vi "Scanning Motion One Direction for Y Multiple Readings per Point With Phase Info.vi"() -> ()   [LabVIEW 2021]
uses:
  <vilib>/Utility/file.llb/Write Delimited Spreadsheet (DBL).vi
  MID-main/Marlin Instrument Driver/Marlin Instrument Driver.lvlib
  <instrlib>/Siglent SDS 1000 2000 Series/Siglent SDS 1000 2000 Series.lvlib
panel:
  in  "Samples per pt":dbl=5.0
  in  "VISA resource name o-scope":refnum<visa-resource-name>="USB0::0xF4ED::0xEE3A::SDS1EDED5R2476::INSTR"
  in  "Measurement (0: Vpp)":u16(ring) items=["Vpp", "Vmax", "Vmin", "Vamp", "Vtop", "Vbase", "Vavg", "Mean", "Vrms", "Crms", "FOV", "FPRE", "ROV", "RPRE", "Period", "Freq", "+Wid", "-Wid", "Rise Time", "Fall Time", "Bwid", "+Duty", "-Duty"]
  in  "Source (1: Channel 1)":u16(ring)=1 items=["Channel 1"=1, "Channel 2"=2, "Channel 3"=3, "Channel 4"=4]
  in  "file path (dialog if empty)":path=path "C:/Users/scoughen/Documents/Printer Controll/Coughenour Programs/Scan Data/LiLens500kHzHighResPhaseScanOrthogonal5SampleAvg0SecDelay3mmOffsetFromTransducerNewAmp9.6Vpp.csv"
  in  "T":dbl
  in  "y Flag":string="Negative"
  in  "x Flag":string="Negative"
  in  "linearF":dbl=1000.0
  in  "E":dbl
  in  "rapidF":dbl=3000.0
  in  "zRes":dbl=0.5
  in  "yRes":dbl=0.5
  in  "xRes":dbl=1.0
  in  "zSize":dbl=80.0
  in  "ySize":dbl=50.0
  in  "xSize":dbl=5.0
  in  "zInit":dbl=149.0
  in  "yInit":dbl=188.0
  in  "xInit":dbl=87.0
  out "error out":errorcluster
  in  "error in (no error)":errorcluster
  in  "VISA resource name":refnum<visa-resource-name>="COM5"
  # "All Units in mm"
  # "Initial Position"
  # "Scan Size"
  # "Scan Resolution"
  # "Extrusion"
  # "Feed Rate"
  # "Read Delay (s)"
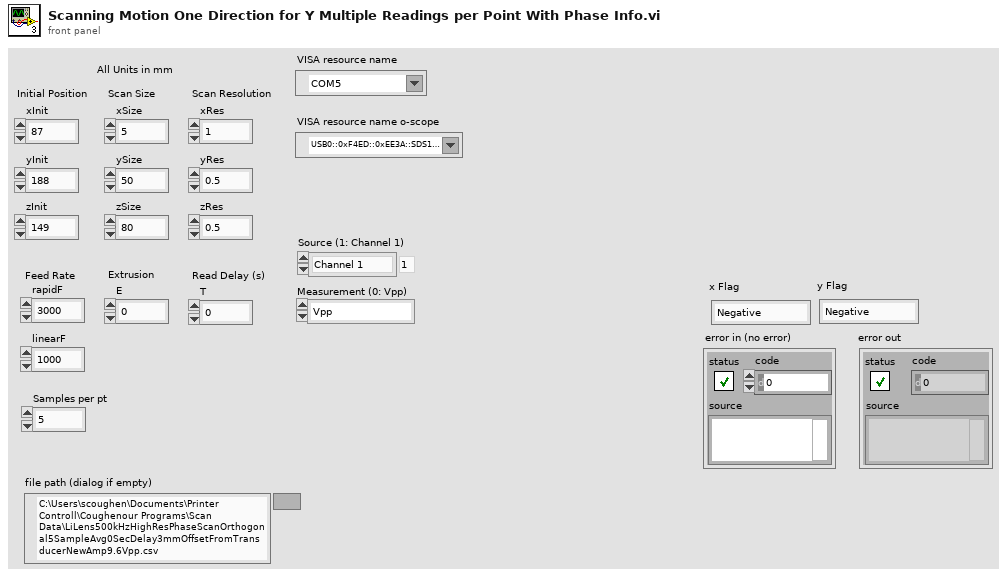
[diagram p1: front panel]
types:
  T1 = cluster{"E":dbl, "rapidF":dbl, "xInit":dbl, "yInit":dbl, "zInit":dbl}
  T2 = cluster{"E":dbl, "linearF":dbl, dbl, "yInit":dbl, "zInit":dbl}
  T3 = cluster{"E":dbl, "linearF":dbl, "xInit":dbl, dbl, "zInit":dbl}
  T4 = cluster{"E":dbl, "linearF":dbl, dbl, "zInit":dbl, "yInit":dbl}
  T5 = cluster{"E":dbl, "linearF":dbl, "xInit":dbl, "yInit":dbl, dbl}
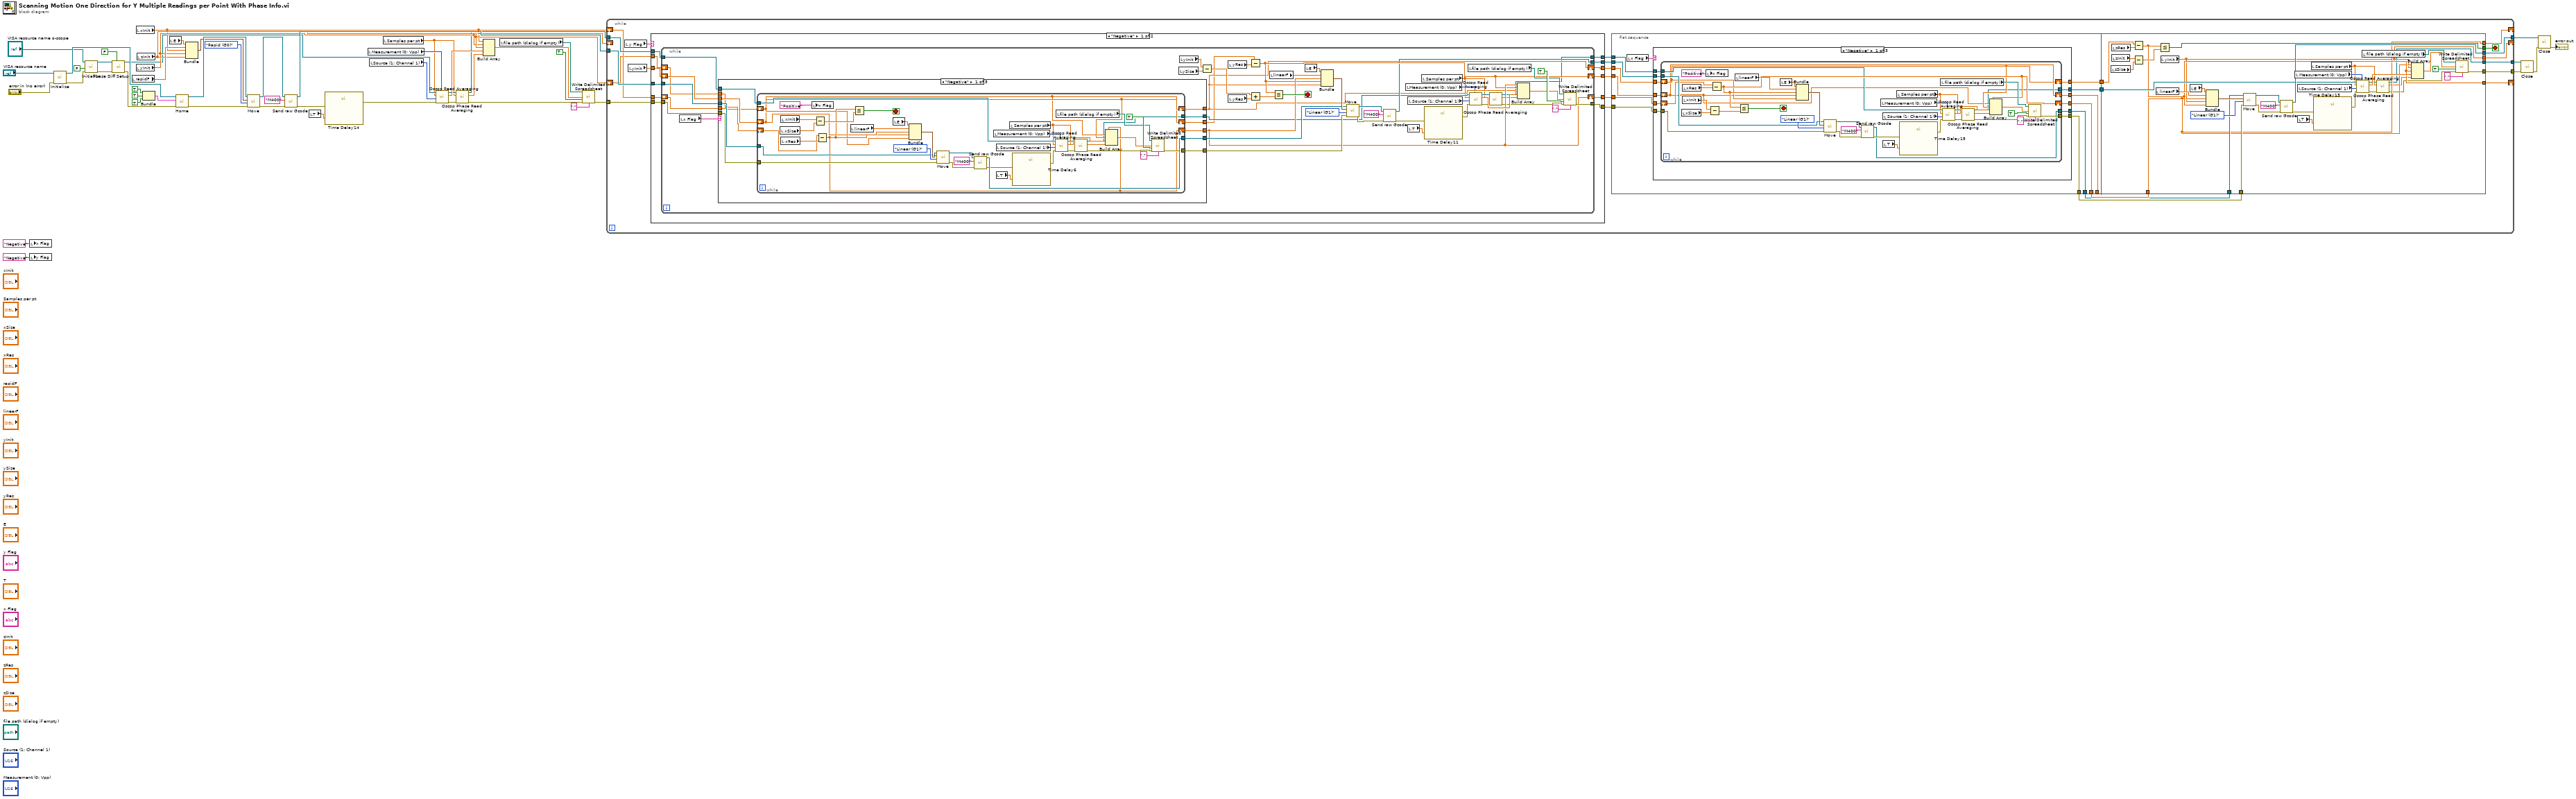
[diagram p0: block diagram]
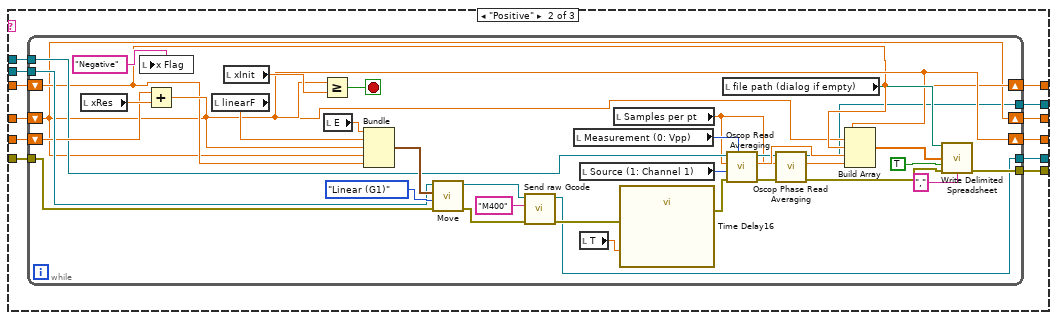
[diagram p2: hidden frame]
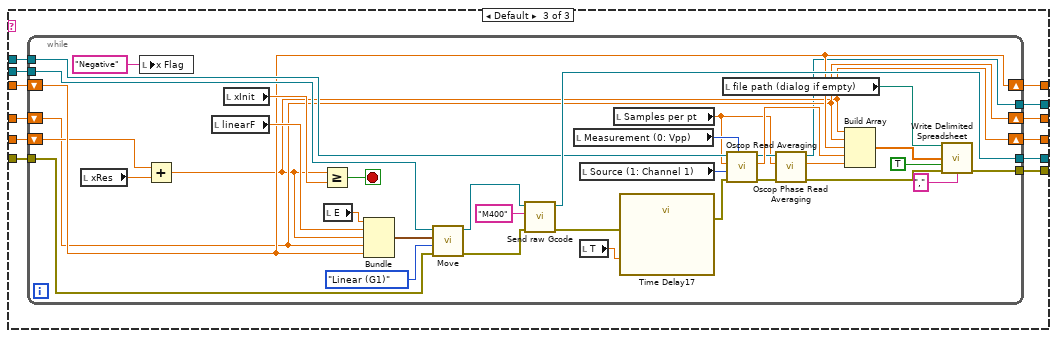
[diagram p3: hidden frame]
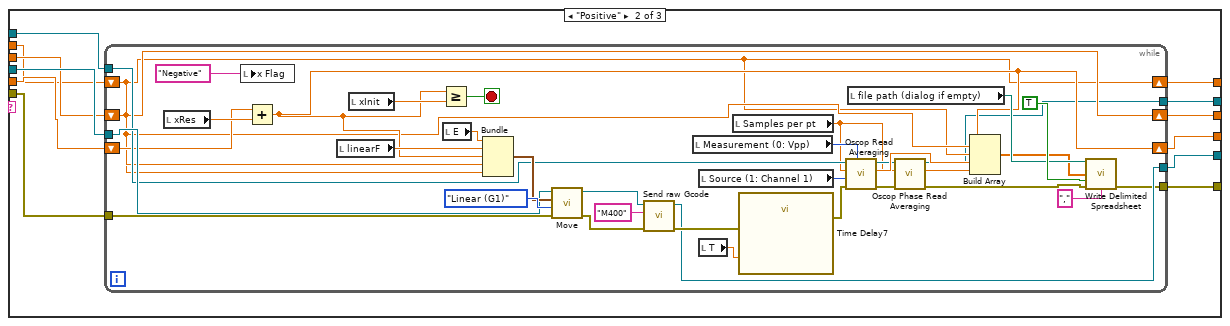
[diagram p4: hidden frame]
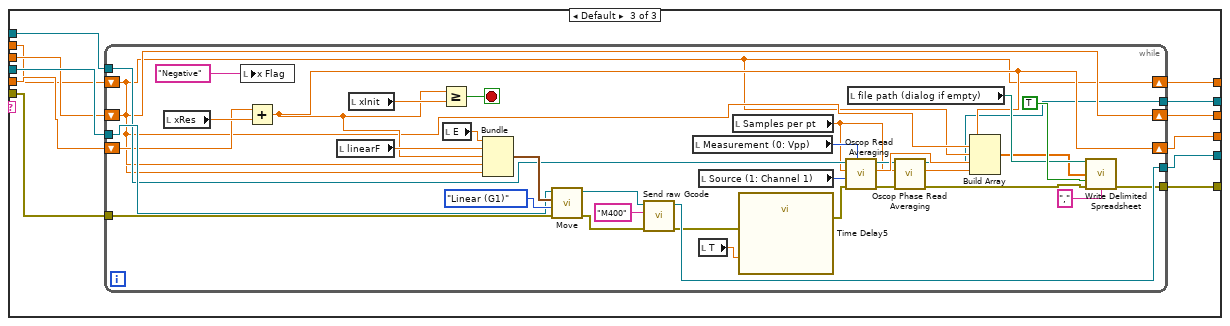
[diagram p5: hidden frame]
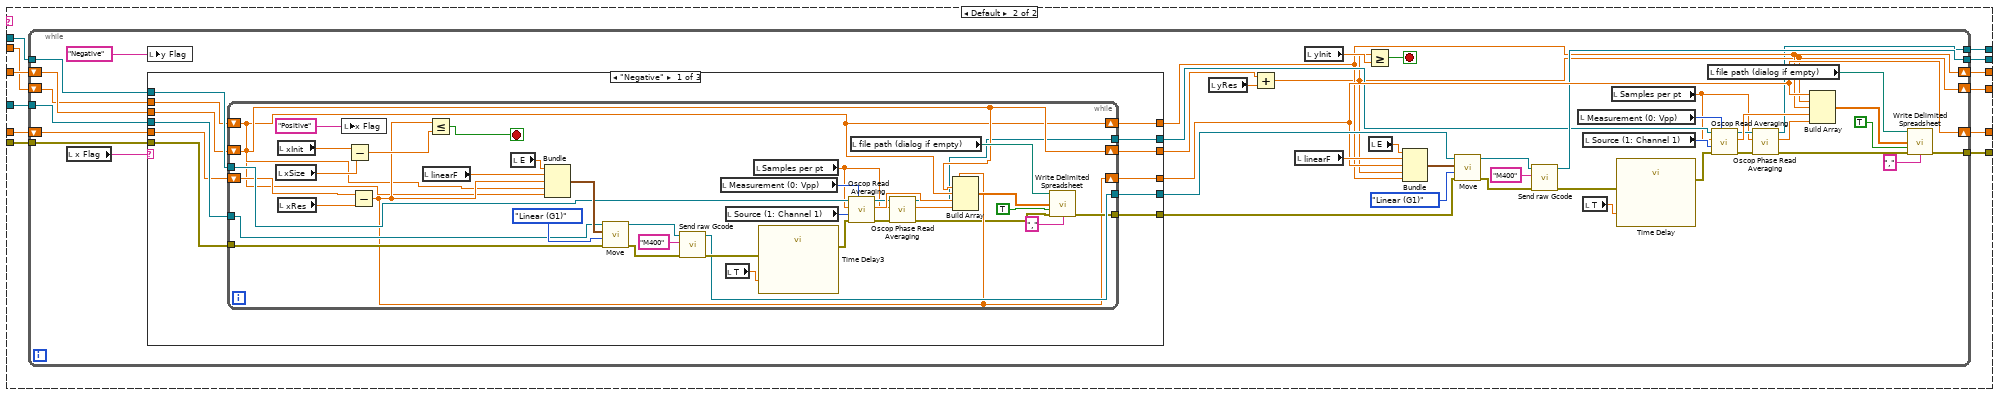
[diagram p6: hidden frame]
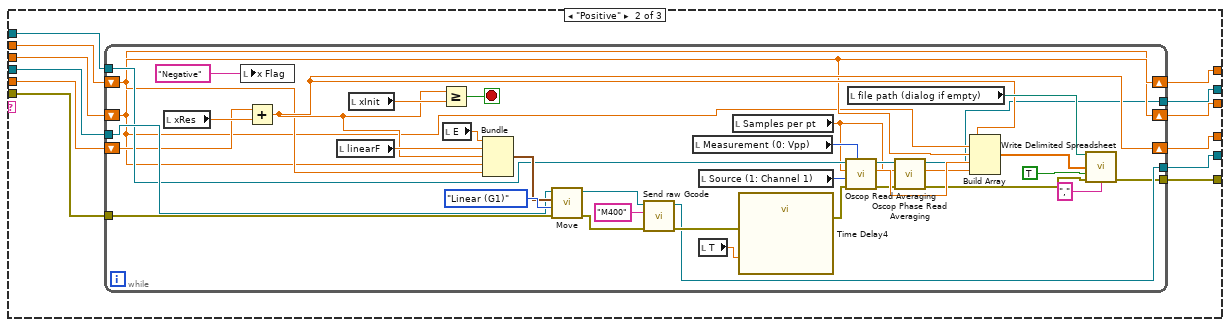
[diagram p7: hidden frame]
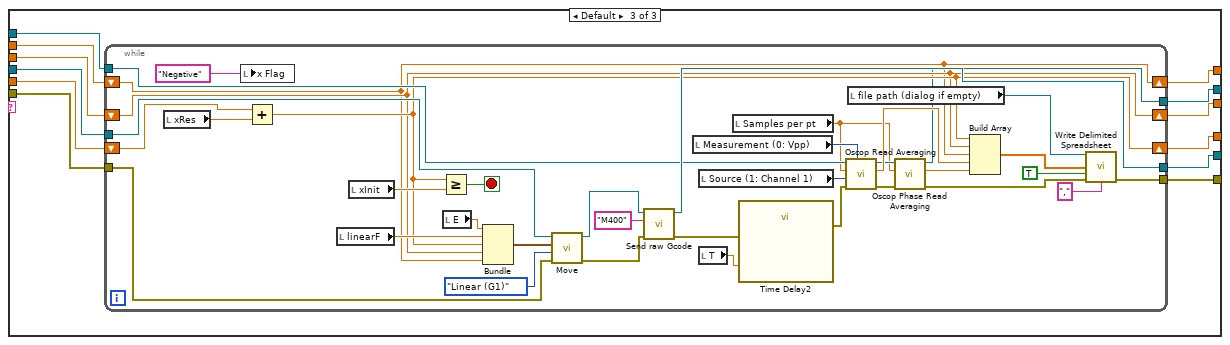
[diagram p8: hidden frame]
diagram:
  n1 = local write "x Flag"("Negative" ("x Flag")) -> ()
  n2 = local write "y Flag"("Negative" ("y Flag")) -> ()
  n3 = call <instrlib>:"Initialize.vi"("error in (no error)"="error in (no error)", "VISA resource name"="VISA resource name") -> ("error out"=w29:errorcluster, "VISA resource name out"=w49:refnum<visa-resource-name>)  [unwired: 8 in]
  n4 = call <instrlib>:"Initialize.vi"("error in (no error)"=w29, "Reset (True)"=FALSE, "VISA resource name"="VISA resource name o-scope") -> ("error out"=w6:errorcluster, "VISA resource name out"=w4:refnum<visa-resource-name>)  [unwired: 7 in]
  n5 = call "Phase Diff Setup.vi"("Perform Auto Setup"=FALSE, "error in (no error)"=w6, "VISA resource name"=w4) -> ("error out"=w5:errorcluster, "VISA resource name out"=w3:refnum<visa-resource-name>)  [unwired: 7 in]
  n6 = local read "rapidF"() -> (w39:dbl)
  n7 = local read "xInit"() -> (w16:dbl)
  n8 = local read "yInit"() -> (w17:dbl)
  n9 = local read "zInit"() -> (w18:dbl)
  n10 = Bundle(TRUE, TRUE, TRUE) -> (w45:cluster{bool, bool, bool})  [unwired: 1 in]
  n11 = local read "E"() -> (w38:dbl)
  n12 = call "Home.vi"("error in (no error)"=w5, "Axes"=w45, "VISA resource name"=w49) -> ("error out"=w44:errorcluster, "VISA resource name out"=w43:refnum<visa-resource-name>)  [unwired: 7 in]
  n13 = Bundle("E"=w38, "rapidF"=w39, "xInit"=w16, "yInit"=w17, "zInit"=w18) -> (w41:T1)  [unwired: 1 in]
  n14 = call "Move.vi"("error in (no error)"=w44, "type"=enum16{"Rapid (G0)", "Linear (G1)"}."Rapid (G0)" ("type 2"), "Distances"=w41, "VISA resource name"=w43) -> ("error out"=w33:errorcluster, "VISA resource name out"=w34:refnum<visa-resource-name>)  [unwired: 6 in]
  n15 = call "Send raw Gcode.vi"("error in (no error)"=w33, "Gcode"="M400", "VISA resource name"=w34) -> ("error out"=w31:errorcluster, "VISA resource name out"=w32:refnum<visa-resource-name>)  [unwired: 5 in, 2 out]
  n16 = local read "T"() -> (w35:dbl)
  n17 = call "Time Delay14"("error in (no error)"=w31, "Delay Time (s)"=w35) -> ("error out"=w21:errorcluster)  [unwired: 9 in]
  n18 = local read "Measurement (0: Vpp)"() -> (w12:u16)
  n19 = local read "Source (1: Channel 1)"() -> (w19:u16)
  n20 = local read "Samples per pt"() -> (w1:dbl)
  n21 = call "Oscop Read Averaging.vi"("Measurement (0: Vpp)"=w12, "error in (no error)"=w21, "Source (1: Channel 1)"=w19, "Numeric in"=w1, "VISA Refnum in"=w3) -> ("error out"=w9:errorcluster, "Numeric out"=w13:dbl, "VISA Refnum out"=w8:refnum<visa-resource-name>)  [unwired: 4 in]
  n22 = call "Oscop Phase Read Averaging.vi"("error in (no error)"=w9, "Numeric in"=w1, "VISA Refnum in"=w8) -> ("error out"=w10:errorcluster, "Numeric out"=w7:dbl, "VISA Refnum out"=w11:refnum<visa-resource-name>)  [unwired: 6 in]
  n23 = Build Array(w16, w17, w18, w13, w7) -> (w22:dbl[])
  n24 = local read "file path (dialog if empty)"() -> (w15:path)
  n25 = call-poly <vilib>:"Write Delimited Spreadsheet.vi"("file path (dialog if empty)"=w15, "1D data"=w22, "append to file? (new file:F)"=TRUE, "error in (no error)"=w10, "delimiter (\\t)"="," ("delimiter (\\t)")) -> ("error out"=w20:errorcluster)  [unwired: 9 in, 1 out]
  n26 = while {
    tunnel: w32 -> [w77]
    tunnel: w20 -> [w76]
    tunnel: [w67] -> w40
    tunnel: [w66] -> w27
    tunnel: [w64] -> w25
    tunnel: w11 -> [w61]
    shift-right: [w56] -> _
    shift-left: w18 -> [w59]
    shift-right: [w55] -> _
    shift-left: w17 -> [_]
    shift-right: [w54] -> _
    shift-left: w16 -> [w60]
    stop <- w65 stop-if-true
    n27 = local read "y Flag"() -> (w75:string)
    n28 = local read "yInit"() -> (w53:dbl)
    n29 = case shown="\"Negative\"" w75 {
      tunnel: w77 -> [w285 w489]
      tunnel: [w282 w488] -> w74
      tunnel: w76 -> [w284 w487]
      tunnel: [w283 w486] -> w73
      tunnel: [w281 w485] -> w71
      tunnel: [w280 w484] -> w72
      tunnel: [w279 w483] -> w58
      tunnel: [w278 w482] -> w62
      tunnel: w61 -> [w277 w481]
      tunnel: w60 -> [w275 w478]
      tunnel: w53 -> [w276 w480]
      tunnel: w59 -> [w274 w479]
      frame "Negative" {
        n30 = while {
          tunnel: w285 -> [w329]
          tunnel: [w300] -> w282
          tunnel: w284 -> [w327]
          tunnel: [w303] -> w283
          tunnel: [w290] -> w278
          tunnel: w277 -> [w298]
          shift-right: [w301] -> w280
          shift-left: w276 -> [w295]
          shift-right: [w302] -> w281
          shift-left: w275 -> [w294]
          shift-right: [w297] -> w279
          shift-left: w274 -> [w293]
          stop <- w325 stop-if-true
          n31 = local read "x Flag"() -> (w324:string)
          n32 = case shown="\"Negative\"" w324 {
            tunnel: w329 -> [w343 w393 w441]
            tunnel: [w340 w392 w440] -> w328
            tunnel: w327 -> [w342 w391 w439]
            tunnel: [w341 w390 w437] -> w326
            tunnel: [w339 w389 w438] -> w302
            tunnel: [w338 w388 w436] -> w296
            tunnel: [w336 w387 w434] -> w299
            tunnel: w298 -> [w337 w386 w435]
            tunnel: w294 -> [w335 w385 w433]
            tunnel: w295 -> [w334 w384 w432]
            tunnel: w293 -> [w332 w383 w431]
            tunnel: [w333 w382 w430] -> w297
            frame "Negative" {
              n33 = while {
                tunnel: w343 -> [w379]
                tunnel: [w366] -> w340
                tunnel: w342 -> [w378]
                tunnel: [w357] -> w341
                tunnel: w337 -> [w356]
                tunnel: [w348] -> w336
                shift-right: [w354] -> w339
                shift-left: w335 -> [w355]
                shift-right: [w352] -> w338
                shift-left: w334 -> [w352]
                shift-right: [w353] -> w333
                shift-left: w332 -> [w353]
                stop <- w377 stop-if-true
                n34 = local read "xSize"() -> (w371:dbl)
                n35 = local read "xInit"() -> (w372:dbl)
                n36 = local read "xRes"() -> (w374:dbl)
                n37 = local write "x Flag"("Positive" ("x Flag")) -> ()
                n38 = Subtract(x=w372, y=w371) -> (x-y=w370:dbl)
                n39 = Subtract(x=w355, y=w374) -> (x-y=w354:dbl)
                n40 = local read "linearF"() -> (w375:dbl)
                n41 = Less Or Equal?(x=w354, y=w370) -> (x <= y?=w377:bool)
                n42 = local read "E"() -> (w376:dbl)
                n43 = Bundle("E"=w376, "linearF"=w375, w354, "yInit"=w352, "zInit"=w353) -> (w380:T2)  [unwired: 1 in]
                n44 = call "Move.vi"("error in (no error)"=w378, "type"=enum16{"Rapid (G0)", "Linear (G1)"}."Linear (G1)" ("type 2"), "Distances"=w380, "VISA resource name"=w379) -> ("error out"=w365:errorcluster, "VISA resource name out"=w367:refnum<visa-resource-name>)  [unwired: 6 in]
                n45 = call "Send raw Gcode.vi"("error in (no error)"=w365, "Gcode"="M400", "VISA resource name"=w367) -> ("error out"=w364:errorcluster, "VISA resource name out"=w366:refnum<visa-resource-name>)  [unwired: 5 in, 2 out]
                n46 = local read "Measurement (0: Vpp)"() -> (w350:u16)
                n47 = local read "Source (1: Channel 1)"() -> (w351:u16)
                n48 = local read "T"() -> (w369:dbl)
                n49 = local read "Samples per pt"() -> (w344:dbl)
                n50 = call "Time Delay6"("error in (no error)"=w364, "Delay Time (s)"=w369) -> ("error out"=w358:errorcluster)  [unwired: 9 in]
                n51 = call "Oscop Read Averaging.vi"("Measurement (0: Vpp)"=w350, "error in (no error)"=w358, "Source (1: Channel 1)"=w351, "Numeric in"=w344, "VISA Refnum in"=w356) -> ("error out"=w345:errorcluster, "Numeric out"=w359:dbl, "VISA Refnum out"=w346:refnum<visa-resource-name>)  [unwired: 4 in]
                n52 = local read "file path (dialog if empty)"() -> (w361:path)
                n53 = call "Oscop Phase Read Averaging.vi"("error in (no error)"=w345, "Numeric in"=w344, "VISA Refnum in"=w346) -> ("error out"=w349:errorcluster, "Numeric out"=w347:dbl, "VISA Refnum out"=w348:refnum<visa-resource-name>)  [unwired: 6 in]
                n54 = Build Array(w354, w352, w353, w359, w347) -> (w360:dbl[])
                n55 = call-poly <vilib>:"Write Delimited Spreadsheet.vi"("file path (dialog if empty)"=w361, "1D data"=w360, "append to file? (new file:F)"=TRUE, "error in (no error)"=w349, "delimiter (\\t)"="," ("delimiter (\\t)")) -> ("error out"=w357:errorcluster)  [unwired: 9 in, 1 out]
              }
            }
            frame "Positive" {
              n56 = while {
                tunnel: w393 -> [w427]
                tunnel: [w414] -> w392
                tunnel: w391 -> [w426]
                tunnel: [w407] -> w390
                tunnel: [w398] -> w387
                tunnel: w386 -> [w405]
                shift-right: [w406] -> w389
                shift-left: w385 -> [w404]
                shift-right: [w403] -> w388
                shift-left: w384 -> [w403]
                shift-right: [w402] -> w382
                shift-left: w383 -> [w402]
                stop <- w425 stop-if-true
                n57 = local read "xRes"() -> (w423:dbl)
                n58 = local write "x Flag"("Negative" ("x Flag")) -> ()
                n59 = Add(x=w404, y=w423) -> (x+y=w406:dbl)
                n60 = local read "linearF"() -> (w422:dbl)
                n61 = local read "xInit"() -> (w424:dbl)
                n62 = Greater Or Equal?(x=w406, y=w424) -> (x >= y?=w425:bool)
                n63 = local read "E"() -> (w421:dbl)
                n64 = Bundle("E"=w421, "linearF"=w422, w406, "yInit"=w403, "zInit"=w402) -> (w428:T2)  [unwired: 1 in]
                n65 = call "Move.vi"("error in (no error)"=w426, "type"=enum16{"Rapid (G0)", "Linear (G1)"}."Linear (G1)" ("type 2"), "Distances"=w428, "VISA resource name"=w427) -> ("error out"=w417:errorcluster, "VISA resource name out"=w415:refnum<visa-resource-name>)  [unwired: 6 in]
                n66 = call "Send raw Gcode.vi"("error in (no error)"=w417, "Gcode"="M400", "VISA resource name"=w415) -> ("error out"=w416:errorcluster, "VISA resource name out"=w414:refnum<visa-resource-name>)  [unwired: 5 in, 2 out]
                n67 = local read "Measurement (0: Vpp)"() -> (w400:u16)
                n68 = local read "Source (1: Channel 1)"() -> (w401:u16)
                n69 = local read "T"() -> (w419:dbl)
                n70 = local read "Samples per pt"() -> (w394:dbl)
                n71 = call "Time Delay7"("error in (no error)"=w416, "Delay Time (s)"=w419) -> ("error out"=w408:errorcluster)  [unwired: 9 in]
                n72 = call "Oscop Read Averaging.vi"("Measurement (0: Vpp)"=w400, "error in (no error)"=w408, "Source (1: Channel 1)"=w401, "Numeric in"=w394, "VISA Refnum in"=w405) -> ("error out"=w396:errorcluster, "Numeric out"=w409:dbl, "VISA Refnum out"=w397:refnum<visa-resource-name>)  [unwired: 4 in]
                n73 = local read "file path (dialog if empty)"() -> (w411:path)
                n74 = call "Oscop Phase Read Averaging.vi"("error in (no error)"=w396, "Numeric in"=w394, "VISA Refnum in"=w397) -> ("error out"=w399:errorcluster, "Numeric out"=w395:dbl, "VISA Refnum out"=w398:refnum<visa-resource-name>)  [unwired: 6 in]
                n75 = Build Array(w406, w403, w402, w409, w395) -> (w410:dbl[])
                n76 = call-poly <vilib>:"Write Delimited Spreadsheet.vi"("file path (dialog if empty)"=w411, "1D data"=w410, "append to file? (new file:F)"=TRUE, "error in (no error)"=w399, "delimiter (\\t)"="," ("delimiter (\\t)")) -> ("error out"=w407:errorcluster)  [unwired: 9 in, 1 out]
              }
            }
            frame Default {
              n77 = while {
                tunnel: w441 -> [w475]
                tunnel: [w464] -> w440
                tunnel: w439 -> [w474]
                tunnel: [w455] -> w437
                tunnel: w435 -> [w454]
                tunnel: [w446] -> w434
                shift-right: [w453] -> w438
                shift-left: w433 -> [w452]
                shift-right: [w451] -> w436
                shift-left: w432 -> [w451]
                shift-right: [w450] -> w430
                shift-left: w431 -> [w450]
                stop <- w473 stop-if-true
                n78 = local read "xRes"() -> (w471:dbl)
                n79 = local write "x Flag"("Negative" ("x Flag")) -> ()
                n80 = Add(x=w452, y=w471) -> (x+y=w453:dbl)
                n81 = local read "linearF"() -> (w470:dbl)
                n82 = local read "xInit"() -> (w472:dbl)
                n83 = Greater Or Equal?(x=w453, y=w472) -> (x >= y?=w473:bool)
                n84 = local read "E"() -> (w469:dbl)
                n85 = Bundle("E"=w469, "linearF"=w470, w453, "yInit"=w451, "zInit"=w450) -> (w476:T2)  [unwired: 1 in]
                n86 = call "Move.vi"("error in (no error)"=w474, "type"=enum16{"Rapid (G0)", "Linear (G1)"}."Linear (G1)" ("type 2"), "Distances"=w476, "VISA resource name"=w475) -> ("error out"=w463:errorcluster, "VISA resource name out"=w465:refnum<visa-resource-name>)  [unwired: 6 in]
                n87 = call "Send raw Gcode.vi"("error in (no error)"=w463, "Gcode"="M400", "VISA resource name"=w465) -> ("error out"=w462:errorcluster, "VISA resource name out"=w464:refnum<visa-resource-name>)  [unwired: 5 in, 2 out]
                n88 = local read "Measurement (0: Vpp)"() -> (w448:u16)
                n89 = local read "Source (1: Channel 1)"() -> (w449:u16)
                n90 = local read "T"() -> (w467:dbl)
                n91 = local read "Samples per pt"() -> (w442:dbl)
                n92 = call "Time Delay5"("error in (no error)"=w462, "Delay Time (s)"=w467) -> ("error out"=w456:errorcluster)  [unwired: 9 in]
                n93 = call "Oscop Read Averaging.vi"("Measurement (0: Vpp)"=w448, "error in (no error)"=w456, "Source (1: Channel 1)"=w449, "Numeric in"=w442, "VISA Refnum in"=w454) -> ("error out"=w444:errorcluster, "Numeric out"=w457:dbl, "VISA Refnum out"=w445:refnum<visa-resource-name>)  [unwired: 4 in]
                n94 = local read "file path (dialog if empty)"() -> (w459:path)
                n95 = call "Oscop Phase Read Averaging.vi"("error in (no error)"=w444, "Numeric in"=w442, "VISA Refnum in"=w445) -> ("error out"=w447:errorcluster, "Numeric out"=w443:dbl, "VISA Refnum out"=w446:refnum<visa-resource-name>)  [unwired: 6 in]
                n96 = Build Array(w453, w451, w450, w457, w443) -> (w458:dbl[])
                n97 = call-poly <vilib>:"Write Delimited Spreadsheet.vi"("file path (dialog if empty)"=w459, "1D data"=w458, "append to file? (new file:F)"=TRUE, "error in (no error)"=w447, "delimiter (\\t)"="," ("delimiter (\\t)")) -> ("error out"=w455:errorcluster)  [unwired: 9 in, 1 out]
              }
            }
          }
          n98 = local read "ySize"() -> (w319:dbl)
          n99 = local read "yInit"() -> (w320:dbl)
          n100 = Subtract(x=w320, y=w319) -> (x-y=w315:dbl)
          n101 = local read "yRes"() -> (w321:dbl)
          n102 = local read "yRes"() -> (w316:dbl)
          n103 = Subtract(x=w296, y=w321) -> (x-y=w301:dbl)
          n104 = Add(x=w315, y=w316) -> (x+y=w317:dbl)
          n105 = local read "linearF"() -> (w322:dbl)
          n106 = Less Or Equal?(x=w301, y=w317) -> (x <= y?=w325:bool)
          n107 = local read "E"() -> (w323:dbl)
          n108 = Bundle("E"=w323, "linearF"=w322, "xInit"=w302, w301, "zInit"=w297) -> (w330:T3)  [unwired: 1 in]
          n109 = call "Move.vi"("error in (no error)"=w326, "type"=enum16{"Rapid (G0)", "Linear (G1)"}."Linear (G1)" ("type 2"), "Distances"=w330, "VISA resource name"=w328) -> ("error out"=w312:errorcluster, "VISA resource name out"=w313:refnum<visa-resource-name>)  [unwired: 6 in]
          n110 = call "Send raw Gcode.vi"("error in (no error)"=w312, "Gcode"="M400", "VISA resource name"=w313) -> ("error out"=w311:errorcluster, "VISA resource name out"=w300:refnum<visa-resource-name>)  [unwired: 5 in, 2 out]
          n111 = local read "Measurement (0: Vpp)"() -> (w292:u16)
          n112 = local read "Source (1: Channel 1)"() -> (w306:u16)
          n113 = local read "T"() -> (w318:dbl)
          n114 = local read "Samples per pt"() -> (w286:dbl)
          n115 = call "Time Delay11"("error in (no error)"=w311, "Delay Time (s)"=w318) -> ("error out"=w304:errorcluster)  [unwired: 9 in]
          n116 = local read "file path (dialog if empty)"() -> (w308:path)
          n117 = call "Oscop Read Averaging.vi"("Measurement (0: Vpp)"=w292, "error in (no error)"=w304, "Source (1: Channel 1)"=w306, "Numeric in"=w286, "VISA Refnum in"=w299) -> ("error out"=w287:errorcluster, "Numeric out"=w305:dbl, "VISA Refnum out"=w288:refnum<visa-resource-name>)  [unwired: 4 in]
          n118 = call "Oscop Phase Read Averaging.vi"("error in (no error)"=w287, "Numeric in"=w286, "VISA Refnum in"=w288) -> ("error out"=w291:errorcluster, "Numeric out"=w289:dbl, "VISA Refnum out"=w290:refnum<visa-resource-name>)  [unwired: 6 in]
          n119 = Build Array(w302, w301, w297, w305, w289) -> (w307:dbl[])
          n120 = call-poly <vilib>:"Write Delimited Spreadsheet.vi"("file path (dialog if empty)"=w308, "1D data"=w307, "append to file? (new file:F)"=TRUE, "error in (no error)"=w291, "delimiter (\\t)"="," ("delimiter (\\t)")) -> ("error out"=w303:errorcluster)  [unwired: 9 in, 1 out]
        }
      }
      frame Default {
        n121 = while {
          tunnel: w489 -> [w530]
          tunnel: [w504] -> w488
          tunnel: w487 -> [w528]
          tunnel: [w506] -> w486
          tunnel: [w494] -> w482
          tunnel: w481 -> [w503]
          shift-right: [w501] -> w483
          shift-left: w480 -> [w500]
          shift-right: [w499] -> w484
          shift-left: w479 -> [w498]
          shift-right: [w505] -> w485
          shift-left: w478 -> [w497]
          stop <- w526 stop-if-true
          n122 = local read "x Flag"() -> (w525:string)
          n123 = local write "y Flag"("Negative" ("y Flag")) -> ()
          n124 = case shown="\"Negative\"" w525 {
            tunnel: w530 -> [w544 w594 w642]
            tunnel: [w541 w593 w641] -> w529
            tunnel: w528 -> [w543 w592 w640]
            tunnel: [w542 w591 w639] -> w527
            tunnel: [w540 w590 w638] -> w505
            tunnel: [w539 w589 w637] -> w518
            tunnel: [w537 w587 w636] -> w502
            tunnel: w503 -> [w538 w588 w635]
            tunnel: [w536 w586 w634] -> w501
            tunnel: w500 -> [w535 w583 w632]
            tunnel: w498 -> [w534 w584 w631]
            tunnel: w497 -> [w533 w585 w633]
            frame "Negative" {
              n125 = while {
                tunnel: w544 -> [w580]
                tunnel: [w565] -> w541
                tunnel: w543 -> [w579]
                tunnel: [w557] -> w542
                tunnel: w538 -> [w559]
                tunnel: [w550] -> w537
                shift-right: [w553] -> w536
                shift-left: w534 -> [w553]
                shift-right: [w556] -> w540
                shift-left: w533 -> [w555]
                shift-right: [w554] -> w539
                shift-left: w535 -> [w554]
                stop <- w578 stop-if-true
                n126 = local read "xSize"() -> (w572:dbl)
                n127 = local read "xInit"() -> (w571:dbl)
                n128 = local read "xRes"() -> (w575:dbl)
                n129 = local write "x Flag"("Positive" ("x Flag")) -> ()
                n130 = Subtract(x=w571, y=w572) -> (x-y=w570:dbl)
                n131 = Subtract(x=w555, y=w575) -> (x-y=w556:dbl)
                n132 = local read "linearF"() -> (w576:dbl)
                n133 = Less Or Equal?(x=w556, y=w570) -> (x <= y?=w578:bool)
                n134 = local read "E"() -> (w577:dbl)
                n135 = Bundle("E"=w577, "linearF"=w576, w556, "yInit"=w554, "zInit"=w553) -> (w581:T2)  [unwired: 1 in]
                n136 = call "Move.vi"("error in (no error)"=w579, "type"=enum16{"Rapid (G0)", "Linear (G1)"}."Linear (G1)" ("type 2"), "Distances"=w581, "VISA resource name"=w580) -> ("error out"=w568:errorcluster, "VISA resource name out"=w566:refnum<visa-resource-name>)  [unwired: 6 in]
                n137 = call "Send raw Gcode.vi"("error in (no error)"=w568, "Gcode"="M400", "VISA resource name"=w566) -> ("error out"=w567:errorcluster, "VISA resource name out"=w565:refnum<visa-resource-name>)  [unwired: 5 in, 2 out]
                n138 = local read "Measurement (0: Vpp)"() -> (w551:u16)
                n139 = local read "Source (1: Channel 1)"() -> (w552:u16)
                n140 = local read "T"() -> (w573:dbl)
                n141 = local read "Samples per pt"() -> (w545:dbl)
                n142 = call "Time Delay3"("error in (no error)"=w567, "Delay Time (s)"=w573) -> ("error out"=w558:errorcluster)  [unwired: 9 in]
                n143 = call "Oscop Read Averaging.vi"("Measurement (0: Vpp)"=w551, "error in (no error)"=w558, "Source (1: Channel 1)"=w552, "Numeric in"=w545, "VISA Refnum in"=w559) -> ("error out"=w547:errorcluster, "Numeric out"=w560:dbl, "VISA Refnum out"=w548:refnum<visa-resource-name>)  [unwired: 4 in]
                n144 = local read "file path (dialog if empty)"() -> (w562:path)
                n145 = call "Oscop Phase Read Averaging.vi"("error in (no error)"=w547, "Numeric in"=w545, "VISA Refnum in"=w548) -> ("error out"=w549:errorcluster, "Numeric out"=w546:dbl, "VISA Refnum out"=w550:refnum<visa-resource-name>)  [unwired: 6 in]
                n146 = Build Array(w556, w554, w553, w560, w546) -> (w561:dbl[])
                n147 = call-poly <vilib>:"Write Delimited Spreadsheet.vi"("file path (dialog if empty)"=w562, "1D data"=w561, "append to file? (new file:F)"=TRUE, "error in (no error)"=w549, "delimiter (\\t)"="," ("delimiter (\\t)")) -> ("error out"=w557:errorcluster)  [unwired: 9 in, 1 out]
              }
            }
            frame "Positive" {
              n148 = while {
                tunnel: w594 -> [w628]
                tunnel: [w615] -> w593
                tunnel: w592 -> [w627]
                tunnel: [w609] -> w591
                tunnel: w588 -> [w607]
                tunnel: [w600] -> w587
                shift-right: [w606] -> w590
                shift-left: w585 -> [w605]
                shift-right: [w604] -> w586
                shift-left: w584 -> [w604]
                shift-right: [w603] -> w589
                shift-left: w583 -> [w603]
                stop <- w626 stop-if-true
                n149 = local read "xRes"() -> (w624:dbl)
                n150 = local write "x Flag"("Negative" ("x Flag")) -> ()
                n151 = Add(x=w605, y=w624) -> (x+y=w606:dbl)
                n152 = local read "linearF"() -> (w623:dbl)
                n153 = local read "xInit"() -> (w625:dbl)
                n154 = Greater Or Equal?(x=w606, y=w625) -> (x >= y?=w626:bool)
                n155 = local read "E"() -> (w622:dbl)
                n156 = Bundle("E"=w622, "linearF"=w623, w606, "yInit"=w603, "zInit"=w604) -> (w629:T2)  [unwired: 1 in]
                n157 = call "Move.vi"("error in (no error)"=w627, "type"=enum16{"Rapid (G0)", "Linear (G1)"}."Linear (G1)" ("type 2"), "Distances"=w629, "VISA resource name"=w628) -> ("error out"=w618:errorcluster, "VISA resource name out"=w616:refnum<visa-resource-name>)  [unwired: 6 in]
                n158 = call "Send raw Gcode.vi"("error in (no error)"=w618, "Gcode"="M400", "VISA resource name"=w616) -> ("error out"=w617:errorcluster, "VISA resource name out"=w615:refnum<visa-resource-name>)  [unwired: 5 in, 2 out]
                n159 = local read "Measurement (0: Vpp)"() -> (w601:u16)
                n160 = local read "Source (1: Channel 1)"() -> (w602:u16)
                n161 = local read "T"() -> (w620:dbl)
                n162 = local read "Samples per pt"() -> (w595:dbl)
                n163 = call "Time Delay4"("error in (no error)"=w617, "Delay Time (s)"=w620) -> ("error out"=w608:errorcluster)  [unwired: 9 in]
                n164 = call "Oscop Read Averaging.vi"("Measurement (0: Vpp)"=w601, "error in (no error)"=w608, "Source (1: Channel 1)"=w602, "Numeric in"=w595, "VISA Refnum in"=w607) -> ("error out"=w597:errorcluster, "Numeric out"=w610:dbl, "VISA Refnum out"=w598:refnum<visa-resource-name>)  [unwired: 4 in]
                n165 = local read "file path (dialog if empty)"() -> (w612:path)
                n166 = call "Oscop Phase Read Averaging.vi"("error in (no error)"=w597, "Numeric in"=w595, "VISA Refnum in"=w598) -> ("error out"=w599:errorcluster, "Numeric out"=w596:dbl, "VISA Refnum out"=w600:refnum<visa-resource-name>)  [unwired: 6 in]
                n167 = Build Array(w606, w603, w604, w610, w596) -> (w611:dbl[])
                n168 = call-poly <vilib>:"Write Delimited Spreadsheet.vi"("file path (dialog if empty)"=w612, "1D data"=w611, "append to file? (new file:F)"=TRUE, "error in (no error)"=w599, "delimiter (\\t)"="," ("delimiter (\\t)")) -> ("error out"=w609:errorcluster)  [unwired: 9 in, 1 out]
              }
            }
            frame Default {
              n169 = while {
                tunnel: w642 -> [w676]
                tunnel: [w665] -> w641
                tunnel: w640 -> [w675]
                tunnel: [w656] -> w639
                tunnel: [w648] -> w636
                tunnel: w635 -> [w655]
                shift-right: [w654] -> w638
                shift-left: w633 -> [w653]
                shift-right: [w652] -> w637
                shift-left: w632 -> [w652]
                shift-right: [w651] -> w634
                shift-left: w631 -> [w651]
                stop <- w674 stop-if-true
                n170 = local read "xRes"() -> (w673:dbl)
                n171 = local write "x Flag"("Negative" ("x Flag")) -> ()
                n172 = Add(x=w653, y=w673) -> (x+y=w654:dbl)
                n173 = local read "linearF"() -> (w672:dbl)
                n174 = local read "xInit"() -> (w668:dbl)
                n175 = Greater Or Equal?(x=w654, y=w668) -> (x >= y?=w674:bool)
                n176 = local read "E"() -> (w671:dbl)
                n177 = Bundle("E"=w671, "linearF"=w672, w654, "yInit"=w652, "zInit"=w651) -> (w677:T2)  [unwired: 1 in]
                n178 = call "Move.vi"("error in (no error)"=w675, "type"=enum16{"Rapid (G0)", "Linear (G1)"}."Linear (G1)" ("type 2"), "Distances"=w677, "VISA resource name"=w676) -> ("error out"=w664:errorcluster, "VISA resource name out"=w666:refnum<visa-resource-name>)  [unwired: 6 in]
                n179 = call "Send raw Gcode.vi"("error in (no error)"=w664, "Gcode"="M400", "VISA resource name"=w666) -> ("error out"=w663:errorcluster, "VISA resource name out"=w665:refnum<visa-resource-name>)  [unwired: 5 in, 2 out]
                n180 = local read "Measurement (0: Vpp)"() -> (w649:u16)
                n181 = local read "Source (1: Channel 1)"() -> (w650:u16)
                n182 = local read "T"() -> (w669:dbl)
                n183 = local read "Samples per pt"() -> (w643:dbl)
                n184 = call "Time Delay2"("error in (no error)"=w663, "Delay Time (s)"=w669) -> ("error out"=w657:errorcluster)  [unwired: 9 in]
                n185 = call "Oscop Read Averaging.vi"("Measurement (0: Vpp)"=w649, "error in (no error)"=w657, "Source (1: Channel 1)"=w650, "Numeric in"=w643, "VISA Refnum in"=w655) -> ("error out"=w644:errorcluster, "Numeric out"=w658:dbl, "VISA Refnum out"=w645:refnum<visa-resource-name>)  [unwired: 4 in]
                n186 = local read "file path (dialog if empty)"() -> (w660:path)
                n187 = call "Oscop Phase Read Averaging.vi"("error in (no error)"=w644, "Numeric in"=w643, "VISA Refnum in"=w645) -> ("error out"=w647:errorcluster, "Numeric out"=w646:dbl, "VISA Refnum out"=w648:refnum<visa-resource-name>)  [unwired: 6 in]
                n188 = Build Array(w654, w652, w651, w658, w646) -> (w659:dbl[])
                n189 = call-poly <vilib>:"Write Delimited Spreadsheet.vi"("file path (dialog if empty)"=w660, "1D data"=w659, "append to file? (new file:F)"=TRUE, "error in (no error)"=w647, "delimiter (\\t)"="," ("delimiter (\\t)")) -> ("error out"=w656:errorcluster)  [unwired: 9 in, 1 out]
              }
            }
          }
          n190 = local read "yRes"() -> (w522:dbl)
          n191 = Add(x=w518, y=w522) -> (x+y=w499:dbl)
          n192 = local read "linearF"() -> (w523:dbl)
          n193 = local read "yInit"() -> (w519:dbl)
          n194 = Greater Or Equal?(x=w499, y=w519) -> (x >= y?=w526:bool)
          n195 = local read "E"() -> (w524:dbl)
          n196 = Bundle("E"=w524, "linearF"=w523, "xInit"=w505, w499, "zInit"=w501) -> (w531:T3)  [unwired: 1 in]
          n197 = call "Move.vi"("error in (no error)"=w527, "type"=enum16{"Rapid (G0)", "Linear (G1)"}."Linear (G1)" ("type 2"), "Distances"=w531, "VISA resource name"=w529) -> ("error out"=w515:errorcluster, "VISA resource name out"=w516:refnum<visa-resource-name>)  [unwired: 6 in]
          n198 = call "Send raw Gcode.vi"("error in (no error)"=w515, "Gcode"="M400", "VISA resource name"=w516) -> ("error out"=w514:errorcluster, "VISA resource name out"=w504:refnum<visa-resource-name>)  [unwired: 5 in, 2 out]
          n199 = local read "Measurement (0: Vpp)"() -> (w496:u16)
          n200 = local read "Source (1: Channel 1)"() -> (w509:u16)
          n201 = local read "T"() -> (w520:dbl)
          n202 = local read "Samples per pt"() -> (w490:dbl)
          n203 = call "Time Delay"("error in (no error)"=w514, "Delay Time (s)"=w520) -> ("error out"=w507:errorcluster)  [unwired: 9 in]
          n204 = local read "file path (dialog if empty)"() -> (w511:path)
          n205 = call "Oscop Read Averaging.vi"("Measurement (0: Vpp)"=w496, "error in (no error)"=w507, "Source (1: Channel 1)"=w509, "Numeric in"=w490, "VISA Refnum in"=w502) -> ("error out"=w491:errorcluster, "Numeric out"=w508:dbl, "VISA Refnum out"=w492:refnum<visa-resource-name>)  [unwired: 4 in]
          n206 = call "Oscop Phase Read Averaging.vi"("error in (no error)"=w491, "Numeric in"=w490, "VISA Refnum in"=w492) -> ("error out"=w495:errorcluster, "Numeric out"=w493:dbl, "VISA Refnum out"=w494:refnum<visa-resource-name>)  [unwired: 6 in]
          n207 = Build Array(w505, w499, w501, w508, w493) -> (w510:dbl[])
          n208 = call-poly <vilib>:"Write Delimited Spreadsheet.vi"("file path (dialog if empty)"=w511, "1D data"=w510, "append to file? (new file:F)"=TRUE, "error in (no error)"=w495, "delimiter (\\t)"="," ("delimiter (\\t)")) -> ("error out"=w506:errorcluster)  [unwired: 9 in, 1 out]
        }
      }
    }
    n209 = flat-sequence {
      tunnel: w74 -> [w89]
      tunnel: w73 -> [w88]
      tunnel: w58 -> [w87]
      tunnel: w72 -> [w86]
      tunnel: w71 -> [w85]
      tunnel: [w84] -> w68
      tunnel: [w83] -> w69
      tunnel: [w82] -> w70
      tunnel: [w81] -> _
      tunnel: [w80] -> w63
      tunnel: w62 -> [w79]
      tunnel: [w78] -> w57
      tunnel: w70 -> [w245]
      tunnel: w69 -> [w265]
      tunnel: w68 -> [w263]
      tunnel: [w249] -> w67
      tunnel: [w257] -> w66
      tunnel: [w258] -> w65
      tunnel: [w241] -> w64
      tunnel: w63 -> [w248]
      tunnel: w57 -> [w247]
      tunnel: [w246] -> w56
      tunnel: [w244] -> w55
      tunnel: [w245] -> w54
      frame #0 {
        n210 = local read "x Flag"() -> (w90:string)
        n211 = case shown="\"Negative\"" w90 {
          tunnel: w89 -> [w102 w152 w200]
          tunnel: [w99 w151 w199] -> w84
          tunnel: w88 -> [w101 w150 w198]
          tunnel: [w100 w149 w196] -> w83
          tunnel: [w98 w148 w197] -> w82
          tunnel: [w97 w147 w195] -> w81
          tunnel: w87 -> [w96 w146 w194]
          tunnel: w86 -> [w91 w145 w189]
          tunnel: w85 -> [w92 w144 w190]
          tunnel: [w95 w143 w193] -> w80
          tunnel: w79 -> [w94 w142 w192]
          tunnel: [w93 w141 w191] -> w78
          frame "Negative" {
            n212 = while {
              tunnel: w102 -> [w138]
              tunnel: [w114] -> w99
              tunnel: w101 -> [w137]
              tunnel: [w119] -> w100
              tunnel: [w108] -> w95
              tunnel: w94 -> [w113]
              shift-right: [w112] -> w93
              shift-left: w96 -> [w112]
              shift-right: [w110] -> w97
              shift-left: w91 -> [w110]
              shift-right: [w118] -> w98
              shift-left: w92 -> [w111]
              stop <- w136 stop-if-true
              n213 = local read "xSize"() -> (w130:dbl)
              n214 = local read "xRes"() -> (w133:dbl)
              n215 = local read "xInit"() -> (w131:dbl)
              n216 = local write "x Flag"("Positive" ("x Flag")) -> ()
              n217 = Subtract(x=w131, y=w130) -> (x-y=w129:dbl)
              n218 = Subtract(x=w111, y=w133) -> (x-y=w118:dbl)
              n219 = local read "linearF"() -> (w134:dbl)
              n220 = Less Or Equal?(x=w118, y=w129) -> (x <= y?=w136:bool)
              n221 = local read "E"() -> (w135:dbl)
              n222 = Bundle("E"=w135, "linearF"=w134, w118, "zInit"=w110, "yInit"=w112) -> (w139:T4)  [unwired: 1 in]
              n223 = call "Move.vi"("error in (no error)"=w137, "type"=enum16{"Rapid (G0)", "Linear (G1)"}."Linear (G1)" ("type 2"), "Distances"=w139, "VISA resource name"=w138) -> ("error out"=w126:errorcluster, "VISA resource name out"=w124:refnum<visa-resource-name>)  [unwired: 6 in]
              n224 = call "Send raw Gcode.vi"("error in (no error)"=w126, "Gcode"="M400", "VISA resource name"=w124) -> ("error out"=w125:errorcluster, "VISA resource name out"=w114:refnum<visa-resource-name>)  [unwired: 5 in, 2 out]
              n225 = local read "Measurement (0: Vpp)"() -> (w109:u16)
              n226 = local read "Source (1: Channel 1)"() -> (w117:u16)
              n227 = local read "T"() -> (w128:dbl)
              n228 = local read "Samples per pt"() -> (w103:dbl)
              n229 = call "Time Delay15"("error in (no error)"=w125, "Delay Time (s)"=w128) -> ("error out"=w116:errorcluster)  [unwired: 9 in]
              n230 = local read "file path (dialog if empty)"() -> (w121:path)
              n231 = call "Oscop Read Averaging.vi"("Measurement (0: Vpp)"=w109, "error in (no error)"=w116, "Source (1: Channel 1)"=w117, "Numeric in"=w103, "VISA Refnum in"=w113) -> ("error out"=w105:errorcluster, "Numeric out"=w115:dbl, "VISA Refnum out"=w104:refnum<visa-resource-name>)  [unwired: 4 in]
              n232 = call "Oscop Phase Read Averaging.vi"("error in (no error)"=w105, "Numeric in"=w103, "VISA Refnum in"=w104) -> ("error out"=w107:errorcluster, "Numeric out"=w106:dbl, "VISA Refnum out"=w108:refnum<visa-resource-name>)  [unwired: 6 in]
              n233 = Build Array(w118, w110, w112, w115, w106) -> (w120:dbl[])
              n234 = call-poly <vilib>:"Write Delimited Spreadsheet.vi"("file path (dialog if empty)"=w121, "1D data"=w120, "append to file? (new file:F)"=TRUE, "error in (no error)"=w107, "delimiter (\\t)"="," ("delimiter (\\t)")) -> ("error out"=w119:errorcluster)  [unwired: 9 in, 1 out]
            }
          }
          frame "Positive" {
            n235 = while {
              tunnel: w152 -> [w186]
              tunnel: [w163] -> w151
              tunnel: w150 -> [w185]
              tunnel: [w168] -> w149
              tunnel: [w158] -> w143
              tunnel: w142 -> [w162]
              shift-right: [w161] -> w141
              shift-left: w146 -> [w161]
              shift-right: [w160] -> w147
              shift-left: w145 -> [w160]
              shift-right: [w167] -> w148
              shift-left: w144 -> [w177]
              stop <- w184 stop-if-true
              n236 = local read "xRes"() -> (w182:dbl)
              n237 = local write "x Flag"("Negative" ("x Flag")) -> ()
              n238 = Add(x=w177, y=w182) -> (x+y=w167:dbl)
              n239 = local read "linearF"() -> (w181:dbl)
              n240 = local read "xInit"() -> (w183:dbl)
              n241 = Greater Or Equal?(x=w167, y=w183) -> (x >= y?=w184:bool)
              n242 = local read "E"() -> (w180:dbl)
              n243 = Bundle("E"=w180, "linearF"=w181, w167, "zInit"=w160, "yInit"=w161) -> (w187:T4)  [unwired: 1 in]
              n244 = call "Move.vi"("error in (no error)"=w185, "type"=enum16{"Rapid (G0)", "Linear (G1)"}."Linear (G1)" ("type 2"), "Distances"=w187, "VISA resource name"=w186) -> ("error out"=w175:errorcluster, "VISA resource name out"=w173:refnum<visa-resource-name>)  [unwired: 6 in]
              n245 = call "Send raw Gcode.vi"("error in (no error)"=w175, "Gcode"="M400", "VISA resource name"=w173) -> ("error out"=w174:errorcluster, "VISA resource name out"=w163:refnum<visa-resource-name>)  [unwired: 5 in, 2 out]
              n246 = local read "Measurement (0: Vpp)"() -> (w159:u16)
              n247 = local read "Source (1: Channel 1)"() -> (w166:u16)
              n248 = local read "T"() -> (w178:dbl)
              n249 = local read "Samples per pt"() -> (w153:dbl)
              n250 = call "Time Delay16"("error in (no error)"=w174, "Delay Time (s)"=w178) -> ("error out"=w165:errorcluster)  [unwired: 9 in]
              n251 = local read "file path (dialog if empty)"() -> (w170:path)
              n252 = call "Oscop Read Averaging.vi"("Measurement (0: Vpp)"=w159, "error in (no error)"=w165, "Source (1: Channel 1)"=w166, "Numeric in"=w153, "VISA Refnum in"=w162) -> ("error out"=w154:errorcluster, "Numeric out"=w164:dbl, "VISA Refnum out"=w155:refnum<visa-resource-name>)  [unwired: 4 in]
              n253 = call "Oscop Phase Read Averaging.vi"("error in (no error)"=w154, "Numeric in"=w153, "VISA Refnum in"=w155) -> ("error out"=w157:errorcluster, "Numeric out"=w156:dbl, "VISA Refnum out"=w158:refnum<visa-resource-name>)  [unwired: 6 in]
              n254 = Build Array(w167, w160, w161, w164, w156) -> (w169:dbl[])
              n255 = call-poly <vilib>:"Write Delimited Spreadsheet.vi"("file path (dialog if empty)"=w170, "1D data"=w169, "append to file? (new file:F)"=TRUE, "error in (no error)"=w157, "delimiter (\\t)"="," ("delimiter (\\t)")) -> ("error out"=w168:errorcluster)  [unwired: 9 in, 1 out]
            }
          }
          frame Default {
            n256 = while {
              tunnel: w200 -> [w234]
              tunnel: [w213] -> w199
              tunnel: w198 -> [w233]
              tunnel: [w217] -> w196
              tunnel: [w205] -> w193
              tunnel: w192 -> [w212]
              shift-right: [w208] -> w197
              shift-left: w190 -> [w210]
              shift-right: [w209] -> w195
              shift-left: w189 -> [w209]
              shift-right: [w211] -> w191
              shift-left: w194 -> [w211]
              stop <- w232 stop-if-true
              n257 = local read "xRes"() -> (w230:dbl)
              n258 = local write "x Flag"("Negative" ("x Flag")) -> ()
              n259 = Add(x=w210, y=w230) -> (x+y=w208:dbl)
              n260 = local read "linearF"() -> (w229:dbl)
              n261 = local read "xInit"() -> (w231:dbl)
              n262 = Greater Or Equal?(x=w208, y=w231) -> (x >= y?=w232:bool)
              n263 = local read "E"() -> (w228:dbl)
              n264 = Bundle("E"=w228, "linearF"=w229, w208, "zInit"=w209, "yInit"=w211) -> (w235:T4)  [unwired: 1 in]
              n265 = call "Move.vi"("error in (no error)"=w233, "type"=enum16{"Rapid (G0)", "Linear (G1)"}."Linear (G1)" ("type 2"), "Distances"=w235, "VISA resource name"=w234) -> ("error out"=w223:errorcluster, "VISA resource name out"=w224:refnum<visa-resource-name>)  [unwired: 6 in]
              n266 = call "Send raw Gcode.vi"("error in (no error)"=w223, "Gcode"="M400", "VISA resource name"=w224) -> ("error out"=w222:errorcluster, "VISA resource name out"=w213:refnum<visa-resource-name>)  [unwired: 5 in, 2 out]
              n267 = local read "Measurement (0: Vpp)"() -> (w207:u16)
              n268 = local read "Source (1: Channel 1)"() -> (w216:u16)
              n269 = local read "T"() -> (w226:dbl)
              n270 = local read "Samples per pt"() -> (w201:dbl)
              n271 = call "Time Delay17"("error in (no error)"=w222, "Delay Time (s)"=w226) -> ("error out"=w214:errorcluster)  [unwired: 9 in]
              n272 = local read "file path (dialog if empty)"() -> (w219:path)
              n273 = call "Oscop Read Averaging.vi"("Measurement (0: Vpp)"=w207, "error in (no error)"=w214, "Source (1: Channel 1)"=w216, "Numeric in"=w201, "VISA Refnum in"=w212) -> ("error out"=w203:errorcluster, "Numeric out"=w215:dbl, "VISA Refnum out"=w202:refnum<visa-resource-name>)  [unwired: 4 in]
              n274 = call "Oscop Phase Read Averaging.vi"("error in (no error)"=w203, "Numeric in"=w201, "VISA Refnum in"=w202) -> ("error out"=w206:errorcluster, "Numeric out"=w204:dbl, "VISA Refnum out"=w205:refnum<visa-resource-name>)  [unwired: 6 in]
              n275 = Build Array(w208, w209, w211, w215, w204) -> (w218:dbl[])
              n276 = call-poly <vilib>:"Write Delimited Spreadsheet.vi"("file path (dialog if empty)"=w219, "1D data"=w218, "append to file? (new file:F)"=TRUE, "error in (no error)"=w206, "delimiter (\\t)"="," ("delimiter (\\t)")) -> ("error out"=w217:errorcluster)  [unwired: 9 in, 1 out]
            }
          }
        }
      }
      frame #1 {
        n277 = local read "zSize"() -> (w261:dbl)
        n278 = local read "zRes"() -> (w259:dbl)
        n279 = local read "zInit"() -> (w260:dbl)
        n280 = Subtract(x=w247, y=w259) -> (x-y=w246:dbl)
        n281 = Subtract(x=w260, y=w261) -> (x-y=w262:dbl)
        n282 = local read "linearF"() -> (w268:dbl)
        n283 = Less Or Equal?(x=w246, y=w262) -> (x <= y?=w258:bool)
        n284 = local read "yInit"() -> (w244:dbl)
        n285 = local read "E"() -> (w269:dbl)
        n286 = Bundle("E"=w269, "linearF"=w268, "xInit"=w245, "yInit"=w244, w246) -> (w267:T5)  [unwired: 1 in]
        n287 = call "Move.vi"("error in (no error)"=w265, "type"=enum16{"Rapid (G0)", "Linear (G1)"}."Linear (G1)" ("type 2"), "Distances"=w267, "VISA resource name"=w263) -> ("error out"=w272:errorcluster, "VISA resource name out"=w271:refnum<visa-resource-name>)  [unwired: 6 in]
        n288 = call "Send raw Gcode.vi"("error in (no error)"=w272, "Gcode"="M400", "VISA resource name"=w271) -> ("error out"=w273:errorcluster, "VISA resource name out"=w249:refnum<visa-resource-name>)  [unwired: 5 in, 2 out]
        n289 = local read "Measurement (0: Vpp)"() -> (w243:u16)
        n290 = local read "Source (1: Channel 1)"() -> (w250:u16)
        n291 = local read "T"() -> (w270:dbl)
        n292 = local read "Samples per pt"() -> (w237:dbl)
        n293 = call "Time Delay13"("error in (no error)"=w273, "Delay Time (s)"=w270) -> ("error out"=w252:errorcluster)  [unwired: 9 in]
        n294 = call "Oscop Read Averaging.vi"("Measurement (0: Vpp)"=w243, "error in (no error)"=w252, "Source (1: Channel 1)"=w250, "Numeric in"=w237, "VISA Refnum in"=w248) -> ("error out"=w239:errorcluster, "Numeric out"=w251:dbl, "VISA Refnum out"=w238:refnum<visa-resource-name>)  [unwired: 4 in]
        n295 = local read "file path (dialog if empty)"() -> (w253:path)
        n296 = call "Oscop Phase Read Averaging.vi"("error in (no error)"=w239, "Numeric in"=w237, "VISA Refnum in"=w238) -> ("error out"=w242:errorcluster, "Numeric out"=w240:dbl, "VISA Refnum out"=w241:refnum<visa-resource-name>)  [unwired: 6 in]
        n297 = Build Array(w245, w244, w246, w251, w240) -> (w254:dbl[])
        n298 = call-poly <vilib>:"Write Delimited Spreadsheet.vi"("file path (dialog if empty)"=w253, "1D data"=w254, "append to file? (new file:F)"=TRUE, "error in (no error)"=w242, "delimiter (\\t)"="," ("delimiter (\\t)")) -> ("error out"=w257:errorcluster)  [unwired: 9 in, 1 out]
      }
    }
  }
  n299 = call "Close.vi"("error in (no error)"=w27, "VISA resource name"=w25) -> ("error out"=w26:errorcluster)  [unwired: 9 in]
  n300 = call "Close.vi"("error in (no error)"=w26, "VISA resource name"=w40) -> ("error out"=→"error out":errorcluster)  [unwired: 9 in]
